vi "Set Tagged Union Info.vi"(7 "application reference (local)":refnum<vi>, 8 "error in (no error)":errorcluster, 9 "Enum Type":variant, 10 "Element Types":variant[](array[variant]), 11 "Variant in":variant) -> (0 "error out":errorcluster, 3 "Variant out":variant)   [LabVIEW 2015, in "Scripting.lvlib"]
uses:
  Scripting.lvlib
  <vilib>/Utility/Data Type/NI_Data Type.lvlib
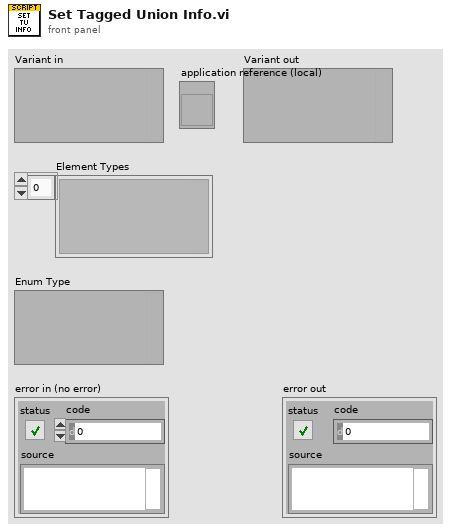
[diagram p1: front panel]
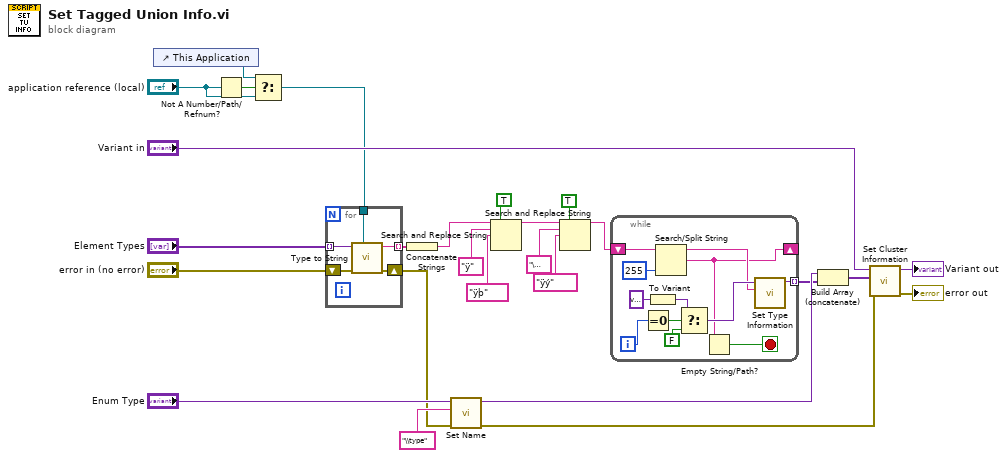
[diagram p0: block diagram]
diagram:
  n1 = control-ref of="This Application"() -> (w3:refnum<vi>)
  n2 = Not A Number/Path/Refnum?(number/path/refnum="application reference (local)") -> (NaN/Path/Refnum?=w4:bool)
  n3 = Select(t=w3, s=w4, f="application reference (local)") -> (s? t:f=w1:refnum<vi>)
  n4 = for {
    tunnel: "Element Types" -> [w31] mode=indexing
    tunnel: [w30] -> w26 mode=indexing
    shift-right: [w28] -> w5
    shift-left: "error in (no error)" -> [w29]
    tunnel: w1 -> [w27]
    n5 = call "Type to String.vi"("application reference (local)"=w27, "Error In"=w29, "Type"=w31) -> ("Error Out"=w28:errorcluster, "String"=w30:string)  [unwired: 7 in]
  }
  n6 = Concatenate Strings(w26) -> (w19:string)
  n7 = call "Set Name.vi"("error in (no error)"=w5, "Name"="\\type", "Type in"="Enum Type") -> ("error out"=w23:errorcluster, "Type out"=w21:variant)  [unwired: 7 in]
  n8 = Search and Replace String(replace all?=TRUE ("replace all? (F)"), input string=w19, search string="ÿ", replace string="ÿþ" ("search string")) -> (result string=w13:string)  [unwired: 4 in, 3 out]
  n9 = Search and Replace String(replace all?=TRUE ("replace all? (F)"), input string=w13, search string="\u0000", replace string="ÿý" ("search string")) -> (result string=w18:string)  [unwired: 4 in, 3 out]
  n10 = while {
    shift-right: [w32] -> _
    shift-left: w18 -> [w43]
    tunnel: [w33] -> w7 mode=indexing
    i -> [w40]
    stop <- w41 stop-if-true
    n11 = Equal To 0?(x=w40) -> (x = 0?=w39:bool)
    n12 = To Variant(anything=variant) -> (Variant=w37:variant)
    n13 = Search/Split String(string=w43, offset (0)=255) -> (substring before match=w34:string, match + rest of string=w32:string)  [unwired: 1 in, 1 out]
    n14 = Select(t=w37, s=w39, f=FALSE) -> (s? t:f=w35:variant)
    n15 = Empty String/Path?(string/path=w32) -> (empty?=w41:bool)
    n16 = call <vilib>:"Set Type Information.vi"("Name"=w34, "Variant in"=w35) -> ("Variant out"=w33:variant)  [unwired: 8 in, 1 out]
  }
  n17 = Build Array (concatenate)(w21, w7) -> (w8:variant[])
  n18 = call <vilib>:"Set Cluster Information.vi"("error in (no error)"=w23, "Cluster Elements"=w8, "Variant in"="Variant in") -> ("error out"=→"error out":errorcluster, "Variant out"=→"Variant out":variant)  [unwired: 7 in]
